vi "Create Radar Plot.vi"() -> (1 "Radar Plot":picture)   [LabVIEW 2011]
doc: "Uses the Radar Plot VI to draw a radar plot in a picture indicator.\n\nNote: You must have the LabVIEW Full or Professional Development Systems to run this example."
panel:
  in  "December data":string[][](table)=[["1", "33", "4", "3", "2", "3"], ["4", "26", "12", "8", "3", "2"], ["2", "12", "2", "14", "4", "3"], ["3", "44", "8", "12", "9", "12"]]
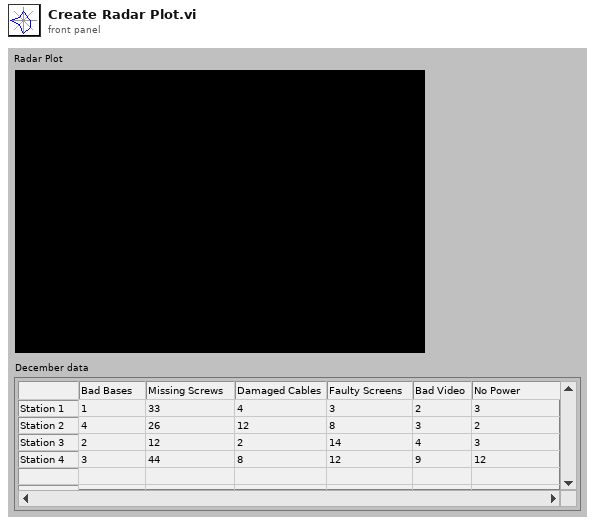
[diagram p1: front panel]
types:
  T1 = cluster{"legend pos (none)":enum16{"none", "top", "right", "bottom", "left"}, "legend text color(white)":u32}
  T2 = cluster{"scale color (black)":u32, "fmt and prec":cluster{"format":enum8{"Decimal", "Scientific", "Engineering", "Binary", "Octal", "Hex"}, "precision":u8}, bool}
  T3 = typedef "LVBoundsTypeDef.ctl" = cluster{"Width":u32, "Height":u32}
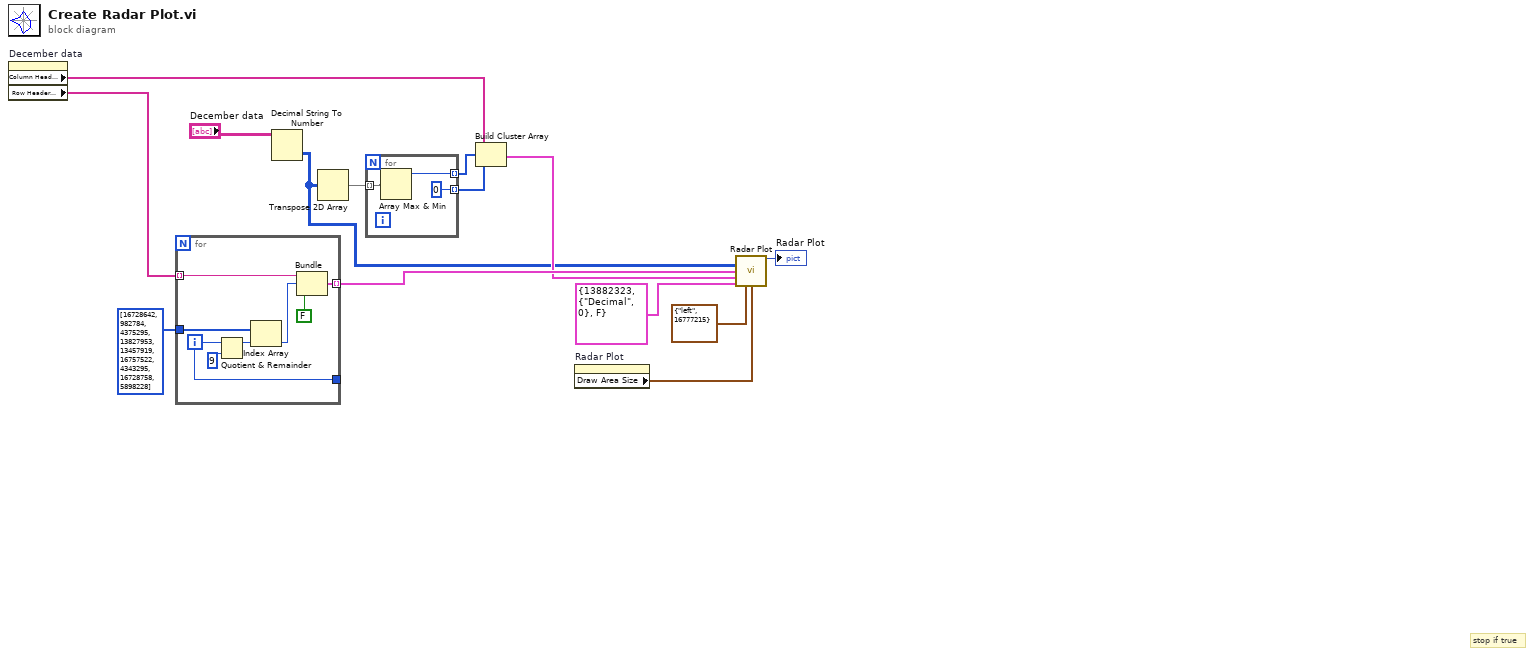
[diagram p0: block diagram]
diagram:
  # "stop if true"
  n1 = property on="December data" class="Tbl (strict)"() -> ("Column Header Strings[]"=w7:string[], "Row Header Strings[]"=w3:string[])  [unwired: 2 in, 2 out]
  n2 = for {
    tunnel: u32[] [16728642, 982784, 4375295, 13827953, 13457919, 16757522, 4343295, 16728758, 5898228] ("Array") -> [w21]
    tunnel: [w18] -> w12 mode=indexing
    tunnel: [w17] -> _
    tunnel: w3 -> [w15] mode=indexing
    i -> [w17]
    n3 = Quotient & Remainder(x=w17, y=9 ("x")) -> (x-y*floor(x/y)=w22:i32)  [unwired: 1 out]
    n4 = Index Array(array=w21, index=w22) -> (element=w19:u32)
    n5 = Bundle(w15, "Plot.Plot Color"=w19, FALSE) -> (w18:cluster{string, "Plot.Plot Color":u32, bool})  [unwired: 1 out]
  }
  n6 = Decimal String To Number(string="December data") -> (number=w1:i32[][])  [unwired: 3 out]
  n7 = Transpose 2D Array(2D array=w1) -> (transposed array=w2:i32[][])
  n8 = for {
    tunnel: w2 -> [w24] mode=indexing
    tunnel: [w23] -> w6 mode=indexing
    tunnel: [0] -> w5 mode=indexing
    n9 = Array Max & Min(array=w24) -> (max value=w23:i32)  [unwired: 3 out]
  }
  n10 = Build Cluster Array(w7, w6, w5) -> (w4:cluster{string, i32, i32}[])
  n11 = property on="Radar Plot" class="Pict"() -> ("Draw Area Size"=w9:T3)  [unwired: 2 in, 2 out]
  n12 = call <vilib>:"Radar Plot.vi"("data"=w1, "plot info"=w12, "axis info"=w4, "axes info"=T2 {"scale color (black)"=13882323, "fmt and prec"={"format"=enum."Decimal", "precision"=0}, FALSE} ("scale info"), "legend info"=T1 {"legend pos (none)"=enum."left", "legend text color(white)"=16777215}, "dimension (w,h)"=w9) -> ("new picture"=→"Radar Plot":picture)  [unwired: 1 in, 8 out]
